vi "sv_Equal Confidence with IC.vi"(0 "scaled signal [EU]":dbl[](array[numeric]) format="%.2f", 1 "BT":dbl format="%.2f", 2 "sampling frequency [Hz]":dbl=10000.0 format="%.2f", 3 "bandwidth [Hz]":dbl format="%.2f", 4 "init/cont (init:F)":bool, 5 "initial filter state":T1 {"peak detector" format="%.2f"; "exponential averaging" format="%.2f"}) -> (6 "exp avg [EU^2 rms] (final value)":dbl format="%.2f", 7 "time constant [ms]":dbl format="%.2f", 8 "final filter state":T1 {"peak detector" format="%.2f"; "exponential averaging" format="%.2f"})   [LabVIEW 2017, in "SoundVib_Octave_2014 standard.lvlib"]
uses:
  <vilib>/addons/Sound and Vibration/svt_Octave/SoundVib_Octave_2014 standard.lvlib
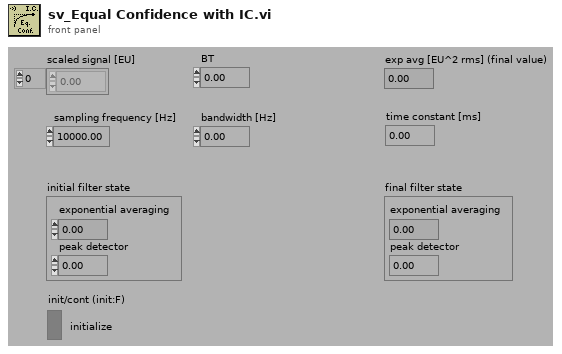
[diagram p1: front panel]
types:
  T1 = cluster{"exponential averaging":dbl, "peak detector":dbl}
  T2 = cluster{"Reverse Coefficients":dbl[], "Forward Coefficients":dbl[]}
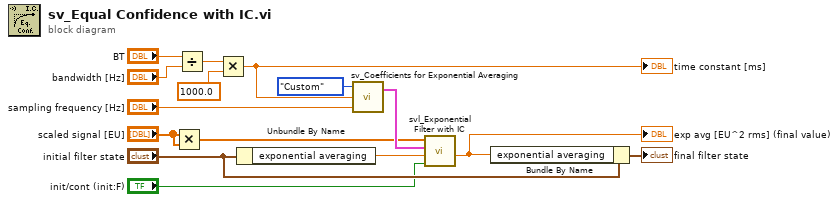
[diagram p0: block diagram]
diagram:
  n1 = Multiply(x="scaled signal [EU]", y="scaled signal [EU]") -> (x*y=w2:dbl[])
  n2 = Divide(x="BT", y="bandwidth [Hz]") -> (x/y=w8:dbl)
  n3 = Multiply(x=w8, y=1000.0) -> (x*y=w9:dbl)
  "time constant [ms]" <- w9
  n4 = Unbundle By Name("initial filter state") -> ("exponential averaging"=w3:dbl)
  n5 = call <vilib>:"sv_Coefficients for Exponential Averaging.vi"("sampling frequency [Hz]"="sampling frequency [Hz]", "time constant [ms]"=w9, "exponential mode"=enum16{"Slow", "Fast", "Impulse", "Custom"}."Custom" ("Mode")) -> ("filter coefficients"=w5:T2)  [unwired: 1 out]
  n6 = call <vilib>:"svl_Exponential Filter with IC.vi"("init/cont (init:F)"="init/cont (init:F)", "initial filter state"=w3, "filter coefficients"=w5, "X"=w2) -> ("final filter state"=w1:dbl)  [unwired: 5 in, 2 out]
  "exp avg [EU^2 rms] (final value)" <- w1
  n7 = Bundle By Name(cluster="initial filter state", "exponential averaging"=w1) -> (→"final filter state":T1)
